vi "Drive Controller.vi"(8 "error in":errorcluster) -> ()   [LabVIEW 2020]
doc: "This VI executes continuously carrying out the current operation and responding to updates or new operation requests. It will often contain the timing or control code that is difficult to place directly in TeleOp. This VI generally opens all sensors and motors and isolates the rest of the robot code from knowing implementation details of how the operations are carried out."
uses:
  <vilib>/Rock Robotics/WPI/Framework/Completion Status.ctl
  Drive Setpoints.ctl
  Drive Operations.ctl
  <vilib>/Rock Robotics/WPI/SafetyOutput/WPI_SafetyOutputConfigMenu.ctl
  <vilib>/Rock Robotics/WPI/RobotDrive/WPI_RobotDriveOpen4MotorWithExistingMotors.vi
  Framework/Robot Global Data.vi
panel:
  in  "Interactive Values":T1
  in  "Buttons":cluster{"Execute Cmd":bool, "Abort Cmd":bool}
  out "Command Timing":cluster{"Start Time (ms)":u32, "Iterations":i32}
  out "Status":T3
  out "Setpoints":T4(graph)
  out "Current\nCmd":string
  # "Tip: The graph shows the motor setpoints. It may also be helpful to observe inputs and sensor values.\nYou may also want to display tuning or debugging controls."
  # "Interactive Command: You may fill in the settings for a command\nand schedule it with the Execute button. You can observe and abort\nany command while fine tuning the code for the controller."
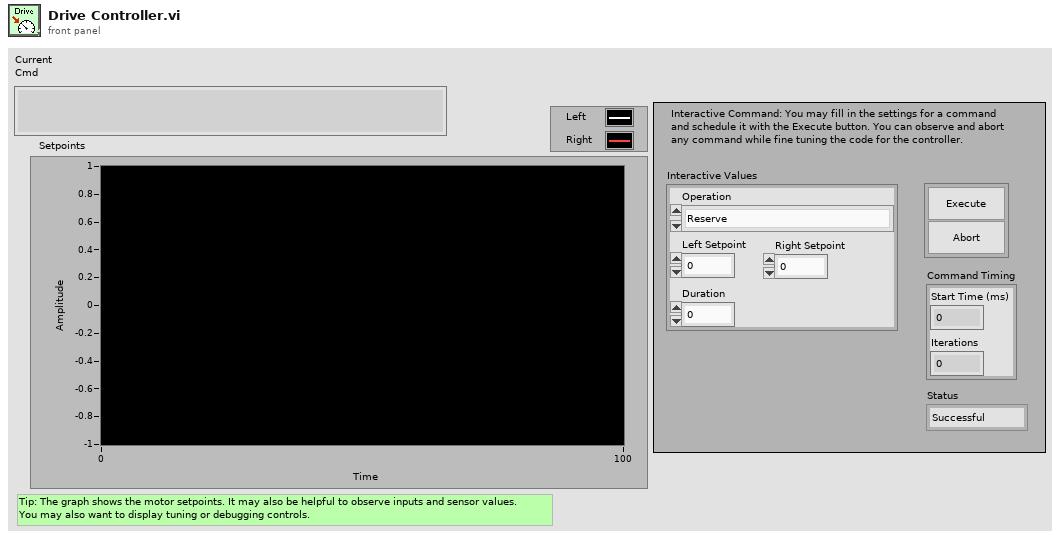
[diagram p1: front panel]
types:
  T1 = typedef "Drive Setpoints.ctl" = cluster{"Operation":T2, "Left Setpoint":dbl, "Right Setpoint":dbl, "Duration":dbl}
  T2 = typedef "Drive Operations.ctl" = enum16{"Reserve", "Read Current", "Immediate", "Drive for Time", "Drive for Distance", "Stop Driving"}
  T3 = typedef "Completion Status.ctl" = enum16{"Successful", "Aborted", "Incomplete"}
  T4 = cluster{"Left Setpoint":dbl, "Right Setpoint":dbl}
  T5 = typedef "WPI_SafetyOutputConfigMenu.ctl" = enum16{"Enable", "Disable"}
  T6 = typedef "WPI_MotorControlDeviceRef.ctl" = cluster{"DeviceStatus":errorcluster, "Type":T7, "PWM":cluster{"PWM Channel":T8, "DeadBand":T9}, "CAN":cluster{"Device Number":u8, "SetOutput VI Ref":variant, "GetOutput VI Ref":variant, "Enable VI Ref":variant, "Disable VI Ref":variant, "Data":variant}, "Invert":bool, "DIO PWM":cluster{"PWM \"Enable\" Channel":T8, "DIOChannel":T10, "PWM Rate":dbl}}
  T7 = typedef "WPI_MotorControlType.ctl" = enum16{"PWM", "CAN", "DIO PWM"}
  T8 = typedef "FPGA_DIOPWMChannel.ctl" = enum8{"PWM 0", "PWM 1", "PWM 2", "PWM 3", "PWM 4", "PWM 5", "PWM 6", "PWM 7", "PWM 8", "PWM 9", "PWM MXP 0", "PWM MXP 1", "PWM MXP 2", "PWM MXP 3", "PWM MXP 4", "PWM MXP 5", "PWM MXP 6", "PWM MXP 7", "PWM MXP 8", "PWM MXP 9", "Invalid"}
  T9 = typedef "WPI_PWMDeadband.ctl" = cluster{"Name":string, "maxPositivePwm":i32, "minPositivePwm":i32, "centerPwm":i32, "maxNegativePwm":i32, "minNegativePwm":i32, "angularRange":u16}
  T10 = typedef "FPGA_DIOChannel.ctl" = enum8{"DIO 0", "DIO 1", "DIO 2", "DIO 3", "DIO 4", "DIO 5", "DIO 6", "DIO 7", "DIO 8", "DIO 9", "DIO MXP 0", "DIO MXP 1", "DIO MXP 2", "DIO MXP 3", "DIO MXP 4", "DIO MXP 5", "DIO MXP 6", "DIO MXP 7", "DIO MXP 8", "DIO MXP 9", "DIO MXP 10", "DIO MXP 11", "DIO MXP 12", "DIO MXP 13", "DIO MXP 14", "DIO MXP 15", "SPI Port CS1", "SPI Port CS2", "SPI Port CS3", "SPI Port MISO", "SPI Port MOSI", "Invalid"}
  T11 = typedef "WPI_RobotDriveDevRef.ctl" = cluster{"DevStatus":errorcluster, "Motors[]":T6[], "Square Inputs":bool, "Max Output":dbl}
  T12 = typedef "Command Status Info.ctl" = cluster{"Name":string, "Status":T3, "notifier out":T13}
  T13 = typedef "Completion Notifier.ctl" = refnum<notifier>
  T14 = cluster{"SubSystem Data":T1, cluster{"Start Time (ms)":u32, "Iterations":i32}, cluster{"Command Info":T12, "Description":string, "Default Command":T1, "queue out":refnum<queue>, "Subsystem Name":string}}
  T15 = cluster{"Don't move motors while reserved":dbl, "Don't move motors while reserved":dbl}
  T16 = cluster{"SubSystem Data":T1, cluster{"Start Time (ms)":u32, "Iterations":i32}, "Default Command Arguments":cluster{"Command Info":T12, "Description":string, "Default Command":T1, "queue out":refnum<queue>, "Subsystem Name":string}}
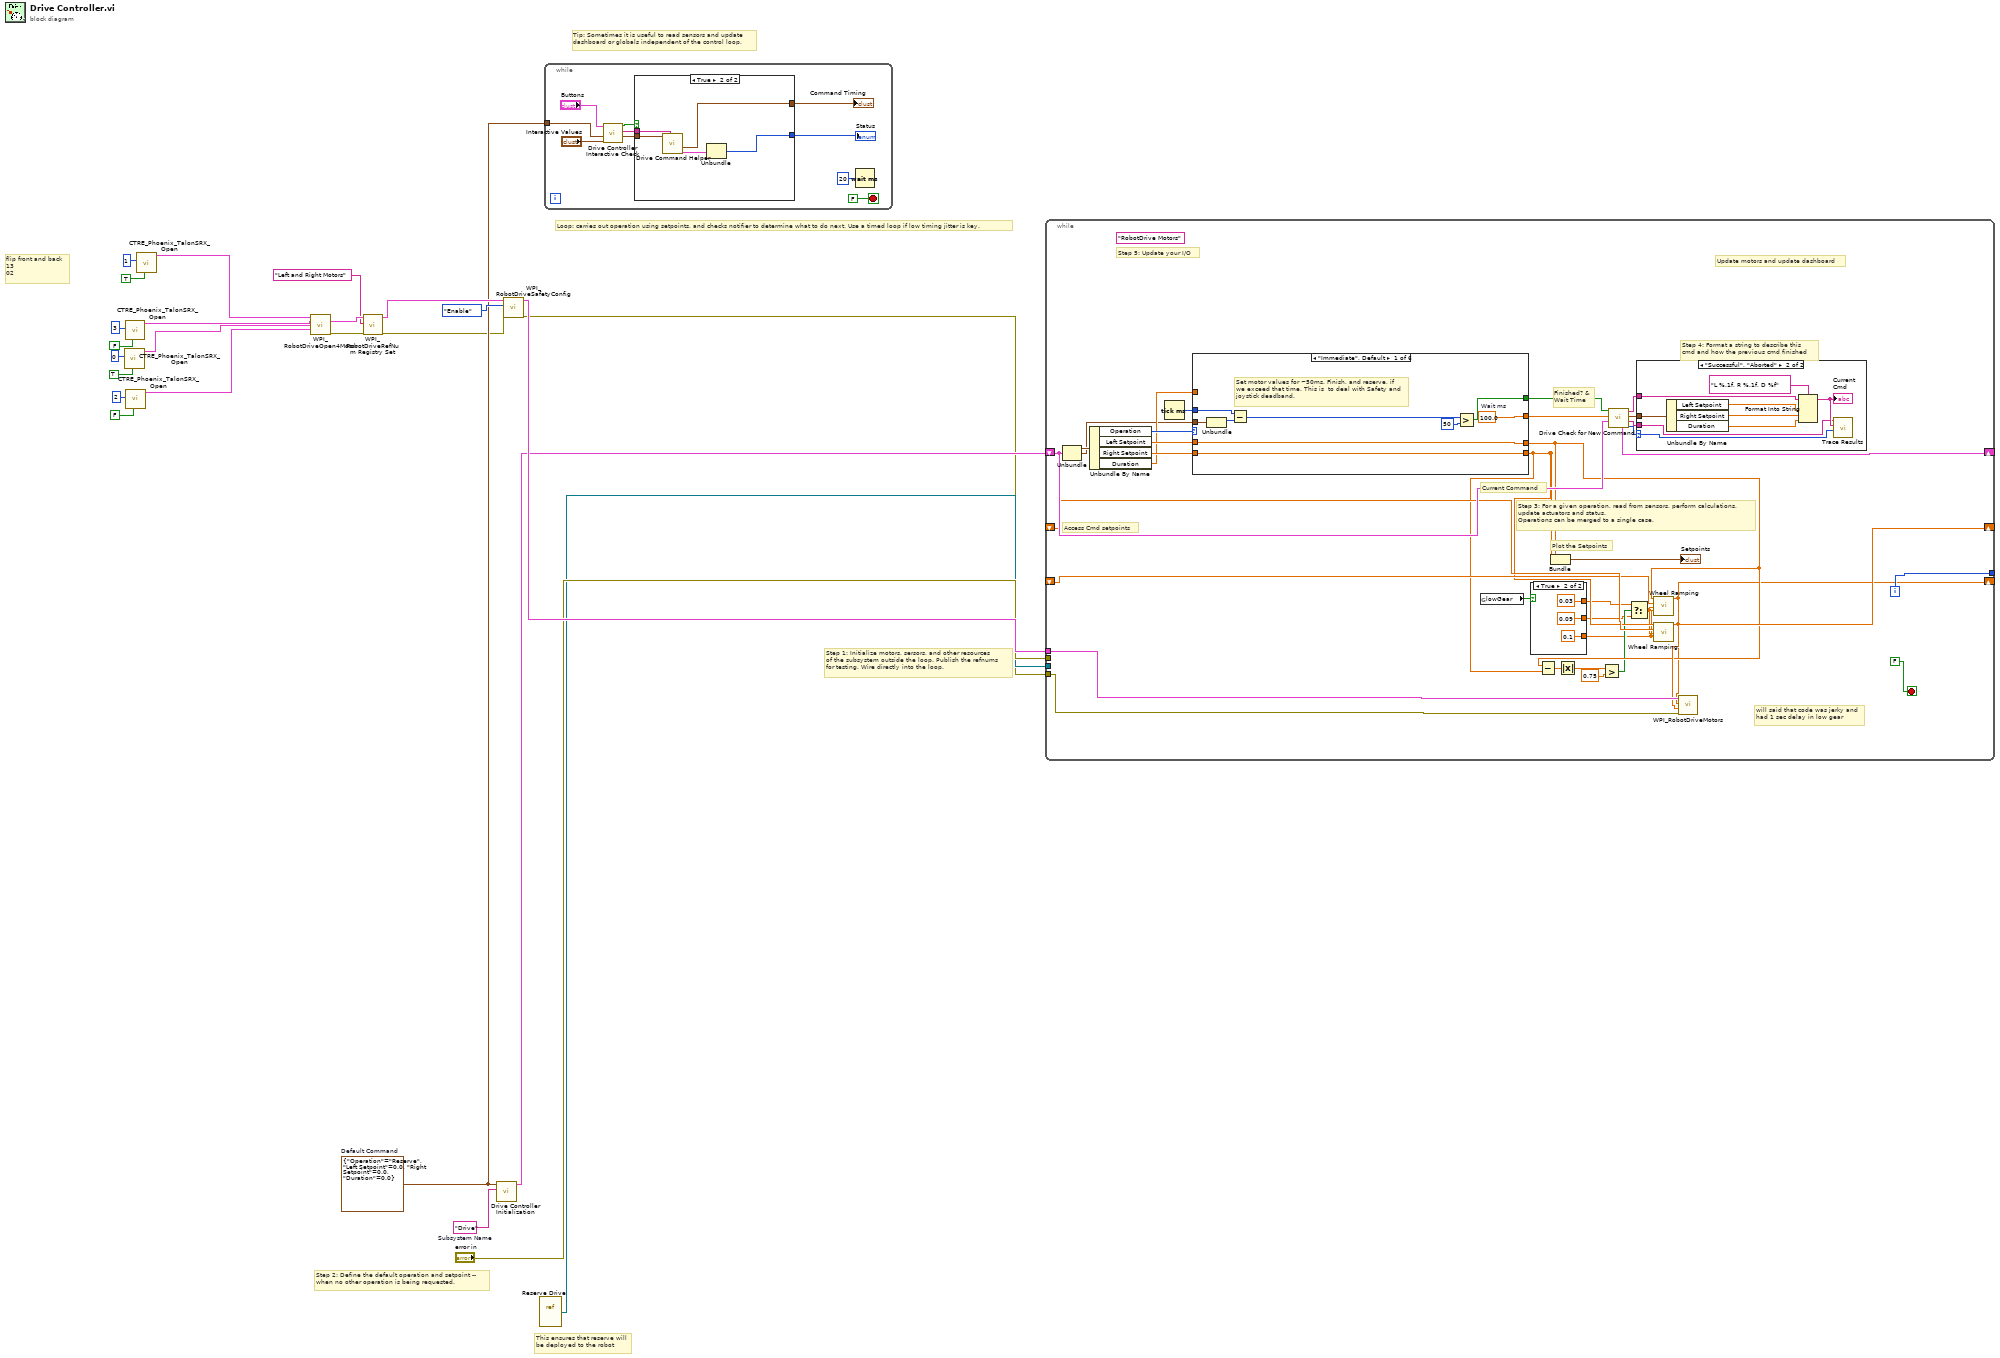
[diagram p0: block diagram]
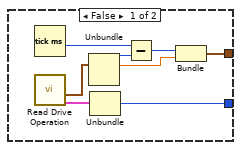
[diagram p2: hidden frame]
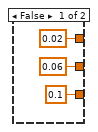
[diagram p3: hidden frame]
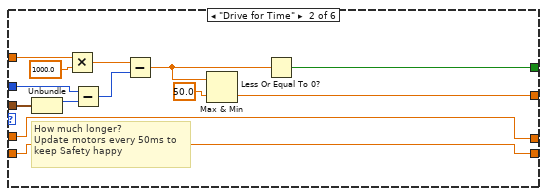
[diagram p5: hidden frame]
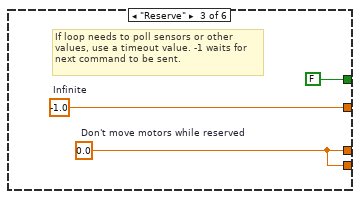
[diagram p6: hidden frame]
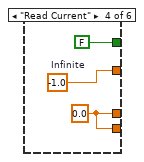
[diagram p7: hidden frame]
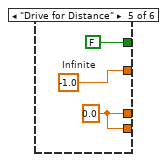
[diagram p8: hidden frame]
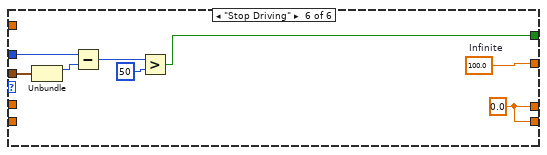
[diagram p9: hidden frame]
diagram:
  w15 = T1 {"Operation"=enum."Reserve", "Left Setpoint"=0.0, "Right Setpoint"=0.0, "Duration"=0.0}  # Default Command
  w25 = "Drive"  # Subsystem Name
  # "flip front and back\n13\n02"
  # "This ensures that reserve will\nbe deployed to the robot"
  # "Tip: Sometimes it is useful to read sensors and update\ndashboard or globals independent of the control loop."
  # "Step 2: Define the default operation and setpoint --\nwhen no other operation is being requested."
  # "Step 1: Initialize motors, sersors, and other resources\nof the subsystem outside the loop. Publish the refnums\nfor testing. Wire directly into the loop."
  # "Loop: carries out operation using setpoints, and checks notifier to determine what to do next. Use a timed loop if low timing jitter is key."
  n1 = call <vilib>:"CTRE_Phoenix_TalonSRX_Open.vi"("Invert"=TRUE, "Device Number"=u8 0) -> ("PhoenixMotorControlDevRef"=w4:T6)  [unwired: 8 in, 1 out]
  n2 = call <vilib>:"CTRE_Phoenix_TalonSRX_Open.vi"("Invert"=FALSE, "Device Number"=u8 3) -> ("PhoenixMotorControlDevRef"=w5:T6)  [unwired: 8 in, 1 out]
  n3 = call <vilib>:"CTRE_Phoenix_TalonSRX_Open.vi"("Invert"=FALSE, "Device Number"=u8 2) -> ("PhoenixMotorControlDevRef"=w3:T6)  [unwired: 8 in, 1 out]
  n4 = call <vilib>:"CTRE_Phoenix_TalonSRX_Open.vi"("Invert"=TRUE, "Device Number"=u8 1) -> ("PhoenixMotorControlDevRef"=w6:T6)  [unwired: 8 in, 1 out]
  n5 = call-poly <vilib>:"WPI_RobotDriveOpen4Motor.vi"("Rear Left Motor Dev Ref"=w6, "Rear Right Motor Dev Ref"=w5, "Front Left Motor Dev Ref"=w4, "Front Right Motor Dev Ref"=w3) -> ("RobotDriveDevRef"=w24:T11, "error out"=w22:errorcluster)  [unwired: 10 in]
  n6 = call <vilib>:"WPI_RobotDriveRefNum Registry Set.vi"("error in (no error)"=w22, "refnum name"="Left and Right Motors", "RobotDriveDevRef"=w24) -> ("error out"=w14:errorcluster, "RobotDriveDevRef"=w21:T11)  [unwired: 1 in, 6 out]
  n7 = call "Drive Controller Initialization.vi"("Subsystem Name"=w25, "Default Command"=w15) -> ("Current Command"=w17:T14)  [unwired: 9 in]
  n8 = call <vilib>:"WPI_RobotDriveSafetyConfig.vi"("error in (no error)"=w14, "mode"=WPI_SafetyOutputConfigMenu."Enable", "RobotDriveDevRef"=w21) -> ("error out"=w13:errorcluster, "RobotDriveDevRef"=w19:T11)  [unwired: 7 in]
  n9 = vi-ref "Reserve Drive.vi"() -> (w16:refnum<vi>)
  n10 = while {
    tunnel: w15 -> [w27]
    stop <- FALSE stop-if-true
    n11 = call "Drive Controller Interactive Check.vi"("Interactive Command In"="Interactive Values", "Default Command"=w27, "Buttons"="Buttons") -> ("Interactive Command Out"=w29:T1, "Trace String"=w30:string, "Schedule"=w31:bool)  [unwired: 6 in]
    n12 = case shown="True" w31 {
      tunnel: [w40 w48] -> w32
      tunnel: [w39 w44] -> w33
      tunnel: w30 -> [_ w46]
      tunnel: w29 -> [_ w45]
      frame False {
        n13 = Tick Count (ms)() -> (millisecond timer value=w43:u32)
        n14 = call "Read Drive Operation.vi"() -> ("Command Info"=w37:T12, "SubSystem Data"=w36:T1)  [unwired: 9 in, 1 out]
        n15 = Unbundle(w36) -> ("Operation"=w41:T2, "Left Setpoint"=w38:dbl)  [unwired: 2 out]
        n16 = Unbundle(w37) -> ("Status"=w40:T3)  [unwired: 2 out]
        n17 = Subtract(x=w43, y=w41) -> (x-y=w42:u32)
        n18 = Bundle(w42, "Left Setpoint"=w38) -> (w39:cluster{u32, "Left Setpoint":dbl})  [unwired: 1 in]
      }
      frame True {
        n19 = call "Drive Command Helper.vi"("Description"=w46, "SubSystem Data"=w45) -> ("Command Info Out"=w47:T12, "Command Timing"=w44:cluster{"Start Time (ms)":u32, "Iterations":i32})  [unwired: 7 in, 1 out]
        n20 = Unbundle(w47) -> ("Status"=w48:T3)  [unwired: 2 out]
      }
    }
    "Status" <- w32
    "Command Timing" <- w33
    n21 = Wait (ms)(milliseconds to wait=u32 20) -> ()  [unwired: 1 out]
  }
  n22 = while {
    shift-right: [w73] -> _
    shift-left: w17 -> [w66]
    tunnel: [w82] -> _
    tunnel: w19 -> [w63]
    tunnel: "error in" -> [_]
    tunnel: w16 -> [_]
    shift-right: [w62] -> _
    shift-left: _ -> [w65]
    shift-right: [w58] -> _
    shift-left: _ -> [w64]
    tunnel: w13 -> [w61]
    i -> [w82]
    stop <- FALSE stop-if-true
    (unwired) "RobotDrive Motors" ("Name")
    # "will said that code was jerky and\nhad 1 sec delay in low gear"
    # "Step 5: Update your I/O"
    # "Step 4: Format a string to describe this\ncmd and how the previous cmd finished"
    # "Current Command"
    # "Update motors and update dashboard"
    # "Plot the Setpoints"
    # "Access Cmd setpoints"
    # "Finished? &\nWait Time"
    # "Step 3: For a given operation, read from sensors, perform calculations,\nupdate actuators and status.\nOperations can be merged to a single case."
    n23 = Unbundle(w66) -> ("SubSystem Data"=w80:T1, w67:cluster{"Start Time (ms)":u32, "Iterations":i32})  [unwired: 1 out]
    n24 = Unbundle By Name(w80) -> ("Operation"=w79:T2, "Left Setpoint"=w78:dbl, "Right Setpoint"=w77:dbl, "Duration"=w76:dbl)
    n25 = Tick Count (ms)() -> (millisecond timer value=w75:u32)
    n26 = case shown="\"Immediate\", Default" w79 {
      tunnel: [w107 w108 w123 w124 w127 w136] -> w72
      tunnel: [w100 w115 FALSE ("ignore previous (F)") FALSE ("ignore previous (F)") FALSE ("ignore previous (F)") w130] -> w71
      tunnel: w67 -> [w99 w117 _ _ _ w131]
      tunnel: [w106 w114 w121 w126 w129 w137] -> w60
      tunnel: [w105 w113 w121 w126 w129 w137] -> w59
      tunnel: w78 -> [w106 w114 _ _ _ _]
      tunnel: w77 -> [w105 w113 _ _ _ _]
      tunnel: w76 -> [_ w112 _ _ _ _]
      tunnel: w75 -> [w101 w111 _ _ _ w132]
      frame "Immediate", Default {
        w107 = 100.0  # Wait ms
        # "Set motor values for ~50ms. Finish, and reserve, if\nwe exceed that time. This is  to deal with Safety and\njoystick deadband."
        n27 = Unbundle(w99) -> ("Start Time (ms)"=w102:u32)  [unwired: 1 out]
        n28 = Subtract(x=w101, y=w102) -> (x-y=w103:u32)
        n29 = Greater?(x=w103, y=u8 50 ("Left Motor")) -> (0:w100:bool)
      }
      frame "Drive for Time" {
        # "How much longer?\nUpdate motors every 50ms to\nkeep Safety happy"
        n30 = Unbundle(w117) -> ("Start Time (ms)"=w116:u32)  [unwired: 1 out]
        n31 = Multiply(x=w112, y=1000.0) -> (x*y=w119:dbl)
        n32 = Subtract(x=w111, y=w116) -> (x-y=w120:u32)
        n33 = Subtract(x=w119, y=w120) -> (x-y=w110:dbl)
        n34 = Max & Min(x=w110, y=50.0) -> (min(x,y)=w108:dbl)  [unwired: 1 out]
        n35 = Less Or Equal To 0?(x=w110) -> (x <= 0?=w115:bool)
      }
      frame "Reserve" {
        w121 = 0.0  # Don't move motors while reserved
        w123 = -1.0  # Infinite
        # "If loop needs to poll sensors or other\nvalues, use a timeout value. -1 waits for\nnext command to be sent."
      }
      frame "Read Current" {
        w124 = -1.0  # Infinite
        w126 = 0.0 ("Don't move motors while reserved")
      }
      frame "Drive for Distance" {
        w127 = -1.0  # Infinite
        w129 = 0.0 ("Don't move motors while reserved")
      }
      frame "Stop Driving" {
        w136 = 100.0  # Infinite
        w137 = 0.0 ("Don't move motors while reserved")
        n36 = Unbundle(w131) -> ("Start Time (ms)"=w133:u32)  [unwired: 1 out]
        n37 = Subtract(x=w132, y=w133) -> (x-y=w134:u32)
        n38 = Greater?(x=w134, y=u8 50 ("Left Motor")) -> (0:w130:bool)
      }
    }
    n39 = global read "Robot Global Data.vi" "lowGear"() -> (w52:bool)
    n40 = case shown="True" w52 {
      tunnel: [0.02 ("t") 0.03 ("t")] -> w51
      tunnel: [0.06 ("MaxRamping") 0.09 ("MaxRamping")] -> w50
      tunnel: [0.1 ("MaxDeceleration") 0.1 ("MaxDeceleration")] -> w49
      frame False {
      }
      frame True {
      }
    }
    n41 = Subtract(x=w60, y=w59) -> (x-y=w55:dbl)
    n42 = Bundle("Don't move motors while reserved"=w60, "Don't move motors while reserved"=w59) -> (→"Setpoints":T15)  [unwired: 1 in]
    n43 = Absolute Value(x=w55) -> (abs(x)=w56:dbl)
    n44 = Greater?(x=w56, y=0.75) -> (0:w57:bool)
    n45 = call "Drive Check for New Command.vi"("input cluster"=w66, "Wait time (ms)"=w72, "Finished?"=w71) -> ("Completion"=w74:T3, "Subsystem Name"=w68:string, "Current Command"=w69:T1, "Initial Trace String"=w70:string, "Next Command"=w73:T16)  [unwired: 4 in]
    n46 = Select(t=w51, s=w57, f=w50) -> (s? t:f=w53:dbl)
    n47 = case shown="\"Successful\", \"Aborted\"" w74 {
      selector: w74 -> [_ w98]
      tunnel: w70 -> [_ w93]
      tunnel: w69 -> [_ w94]
      tunnel: w68 -> [_ w90]
      frame "Incomplete", Default {
        # "Continuing current command"
      }
      frame "Successful", "Aborted" {
        # "Report and setup for next command"
        n48 = Unbundle By Name(w94) -> ("Left Setpoint"=w96:dbl, "Right Setpoint"=w97:dbl, "Duration"=w91:dbl)
        n49 = Format Into String(format string="L %.1f, R %.1f, D %f", initial string=w93, w96, w97, w91) -> (resulting string=w92:string)  [unwired: 1 in, 1 out]
        "Current\nCmd" <- w92
        n50 = call <vilib>:"Trace Results.vi"("Status of previous command"=w98, "Description"=w92, "Subsystem"=w90) -> ()  [unwired: 9 in]
      }
    }
    n51 = call "Wheel Ramping.vi"("Joystick Value"=w60, "Current Value"=w64, "MaxRamping"=w53, "MaxDeceleration"=w49) -> ("Changed Speed"=w58:dbl)  [unwired: 11 in]
    n52 = call "Wheel Ramping.vi"("Joystick Value"=w59, "Current Value"=w65, "MaxRamping"=w53, "MaxDeceleration"=w49) -> ("Changed Speed"=w62:dbl)  [unwired: 11 in]
    n53 = call <vilib>:"WPI_RobotDriveMotors.vi"("error in (no error)"=w61, "RightSpeed"=w62, "LeftSpeed"=w58, "RobotDriveDevRef"=w63) -> ()  [unwired: 5 in, 3 out]
  }
